vi "Tree_GetChildren.vi"(8 "Error In":errorcluster, 10 "Parent Tag":string, 11 "Tree Refnum IN":refnum<vi>) -> (0 "Error Out":errorcluster, 2 "Children Tags":string[](array[string]), 3 "Tree Refnum OUT":refnum<vi>)   [LabVIEW 2012]
doc: "Gets an array of children tags for a given parent tag.\n\nNote that, to get the tags of grandchildren, this function needs to be called again with the child as the parent tag input."
panel:
  in  "Tree":string(tree)
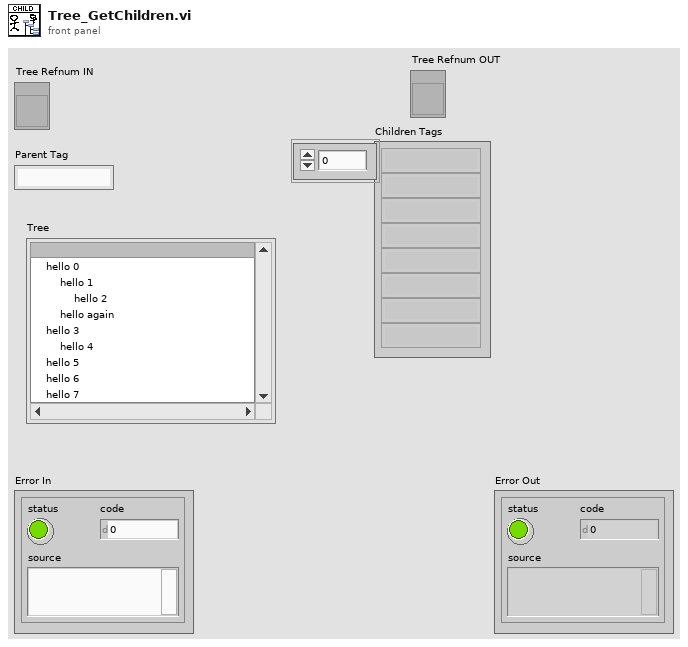
[diagram p1: front panel]
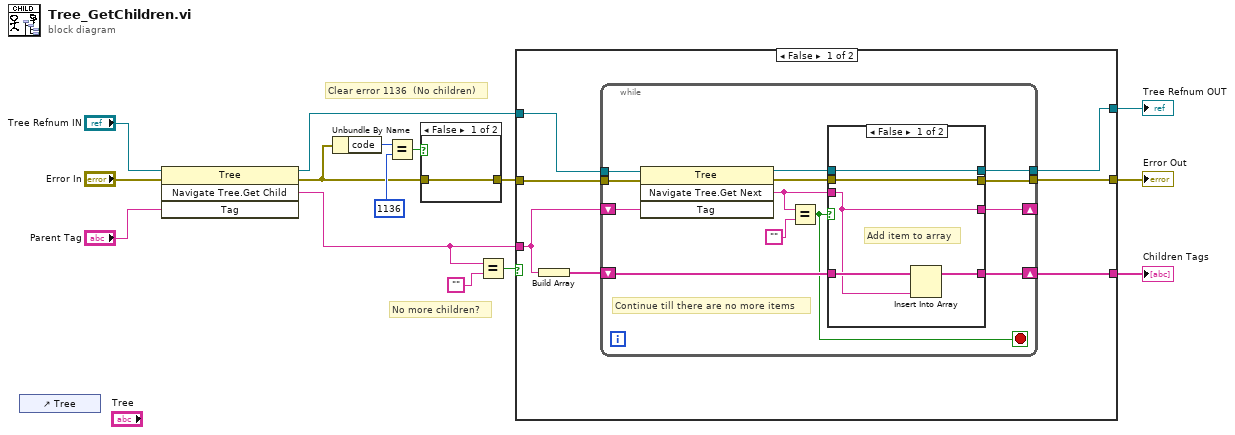
[diagram p0: block diagram]
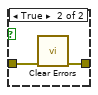
[diagram p2: hidden frame]
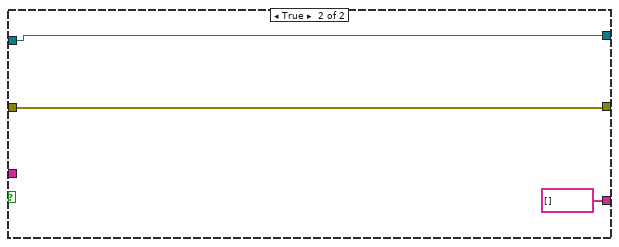
[diagram p4: hidden frame]
diagram:
  # "No more children?"
  # "Clear error 1136  (No children)"
  n1 = control-ref of="Tree"() -> ()  [unwired: 1 out]
  n2 = invoke class="Tree" method="Navigate Tree.Get Child"(reference="Tree Refnum IN", error in="Error In", "Tag"="Parent Tag") -> (reference out=w15:refnum<vi>, error out=w5:errorcluster, "Navigate Tree:Get Child"=w10:string)  [unwired: 1 in, 1 out]
  n3 = Unbundle By Name(w5) -> ("code"=w8:i32)
  n4 = Equal?(x=w8, y=1136) -> (x = y?=w6:bool)
  n5 = case shown="False" w6 {
    tunnel: w5 -> [w16 w18]
    tunnel: [w16 w17] -> w4
    frame False {
    }
    frame True {
      n6 = call <vilib>:"Clear Errors.vi"("error in (no error)"=w18) -> ("error out"=w17:errorcluster)  [unwired: 6 in]
    }
  }
  n7 = Equal?(x=w10, y="") -> (x = y?=w9:bool)
  n8 = case shown="False" w9 {
    tunnel: w4 -> [w25 w50]
    tunnel: w15 -> [w24 w49]
    tunnel: w10 -> [w22 _]
    tunnel: [w21 string[] []] -> w13
    tunnel: [w20 w50] -> w2
    tunnel: [w19 w49] -> w1
    frame False {
      n9 = Build Array(w22) -> (w23:string[])
      n10 = while {
        tunnel: w24 -> [w38]
        tunnel: w25 -> [w37]
        shift-right: [w33] -> w21
        shift-left: w23 -> [w34]
        tunnel: [w30] -> w19
        tunnel: [w29] -> w20
        shift-right: [w26] -> _
        shift-left: w22 -> [w35]
        stop <- w28 stop-if-true
        # "Continue till there are no more items"
        n11 = invoke class="Tree" method="Navigate Tree.Get Next"(reference=w38, error in=w37, "Tag"=w35) -> (reference out=w32:refnum<vi>, error out=w31:errorcluster, "Navigate Tree:Get Next Item"=w27:string)  [unwired: 1 in, 1 out]
        n12 = Equal?(x=w27, y="") -> (x = y?=w28:bool)
        n13 = case shown="False" w28 {
          tunnel: w27 -> [w39 w44]
          tunnel: w34 -> [w43 w47]
          tunnel: [w42 w47] -> w33
          tunnel: w32 -> [w40 w46]
          tunnel: w31 -> [w41 w45]
          tunnel: [w40 w46] -> w30
          tunnel: [w41 w45] -> w29
          tunnel: [w39 w44] -> w26
          frame False {
            # "Add item to array"
            n14 = Insert Into Array(array=w43, new element=w39) -> (w42:string[])  [unwired: 1 in]
          }
          frame True {
          }
        }
      }
    }
    frame True {
    }
  }
  "Error Out" <- w2
  "Children Tags" <- w13
  "Tree Refnum OUT" <- w1
